vi "ITCReplytoDSC.vi"(8 "error in (no error)":errorcluster, 10 "Response":T1) -> (0 "error out":errorcluster)   [LabVIEW 2016]
uses:
  <instrlib>/Mercury iXX/Public/Controls/Response String.ctl
  <instrlib>/Mercury iXX/Mercury iXX.lvlib
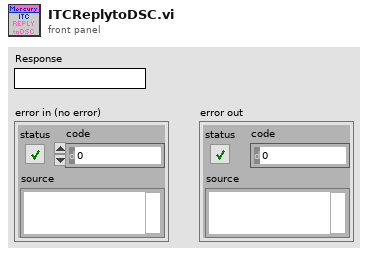
[diagram p1: front panel]
types:
  T1 = typedef "Mercury iXX.lvlib/Response String.ctl" = string
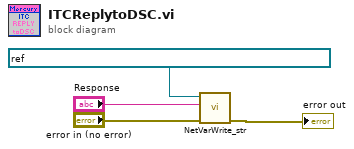
[diagram p0: block diagram]
diagram:
  n1 = call "NetVarWrite_str.vi"("error in (no error)"="error in (no error)", "String"="Response", "Refnum in"=refnum<k21> "ni.var.psp://housesoftheholy/MNK_18T/1820_ITC_Reply") -> ("error out"=→"error out":errorcluster)  [unwired: 8 in]
